vi "AppendConstWfm.vi"(8 "sChnUnit":string="Volts", 9 "sChnName":string="Cal Load", 10 "Nominal Calibration Load (Volts)":dbl format="%.3g", 11 "aWfmsIn":waveform(dbl)[](array[waveform])) -> (3 "aWfmsApndOt":waveform(dbl)[](array[waveform]))   [LabVIEW 2017]
uses:
  <vilib>/Waveform/WDTOps.llb/WDT Index Channel DBL.vi
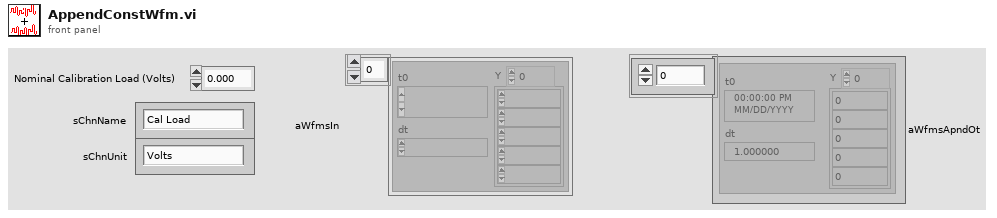
[diagram p1: front panel]
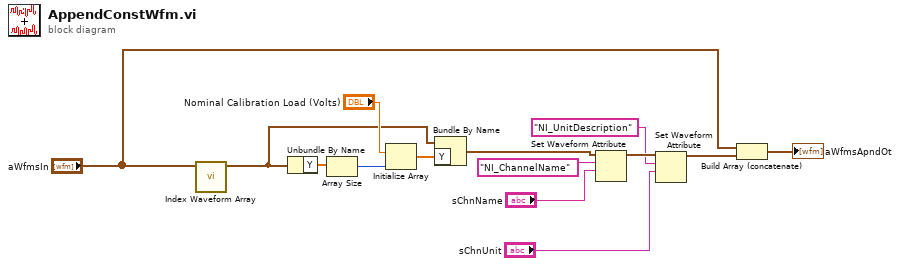
[diagram p0: block diagram]
diagram:
  n1 = call-poly <vilib>:"Index Waveform Array.vi"("waveform array"="aWfmsIn") -> ("waveform"=w4:waveform(dbl))  [unwired: 9 in, 1 out]
  n2 = Unbundle By Name(w4) -> ("Y"=w14:dbl[])
  n3 = Array Size(array=w14) -> (size(s)=w12:i32)
  n4 = Initialize Array("Nominal Calibration Load (Volts)", w12) -> (w13:dbl[])
  n5 = Bundle By Name(cluster=w4, "Y"=w13) -> (w7:waveform(dbl))
  n6 = Set Waveform Attribute(5:"sChnName", 6:"NI_ChannelName" ("name"), 7:w7) -> (3:w9:waveform(dbl))  [unwired: 1 in, 2 out]
  n7 = Set Waveform Attribute(5:"sChnUnit", 6:"NI_UnitDescription" ("name"), 7:w9) -> (3:w3:waveform(dbl))  [unwired: 1 in, 2 out]
  n8 = Build Array (concatenate)("aWfmsIn", w3) -> (→"aWfmsApndOt":waveform(dbl)[])
